vi "CM-TDT-Save config.vi"(0 "configuration file path":path=path "C:/PXI Connections.txt", 5 "Tables":cluster{"Table":T1[]}[](array[cluster]), 9 "Endpoints":cluster{"Items":string[]}[](array[cluster]), 11 "error in (no error)":errorcluster) -> (15 "error out":errorcluster)   [LabVIEW 2015]
uses:
  Type Defs/CM-Connection.ctl
  <vilib>/Utility/config.llb/Write Key (String).vi
  <vilib>/Utility/config.llb/NI_LVConfig.lvlib
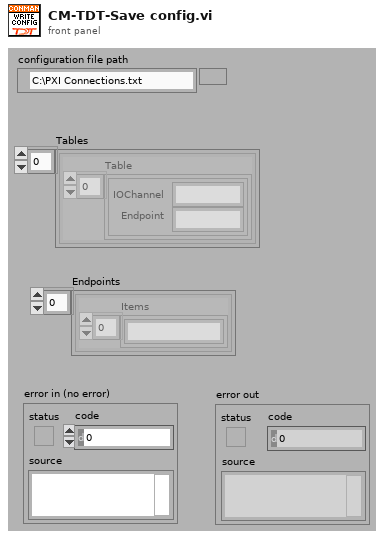
[diagram p1: front panel]
types:
  T1 = typedef "CM-Connection.ctl" = cluster{"IOChannel":string, "Endpoint":string}
  T2 = typedef "NI_LVConfig.lvlib/Config Data RefNum.ctl" = refnum<k1>
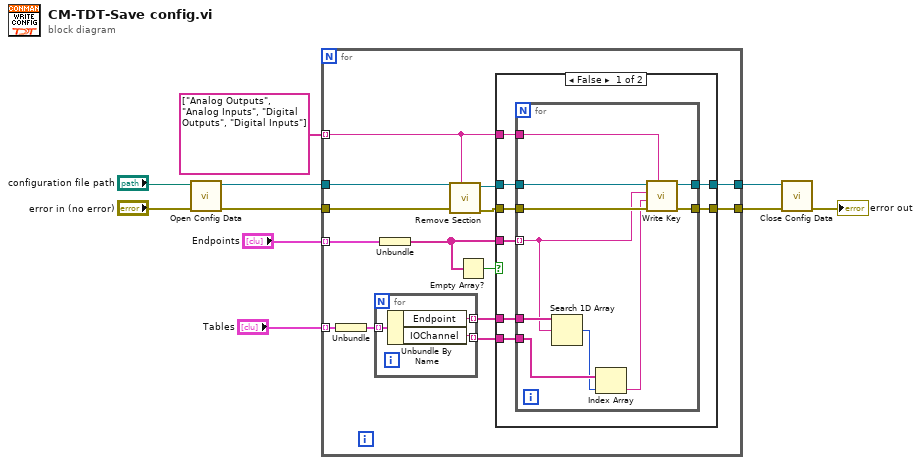
[diagram p0: block diagram]
diagram:
  n1 = call <vilib>:"Open Config Data.vi"("error in (no error)"="error in (no error)", "configuration file path"="configuration file path") -> ("error out"=w5:errorcluster, "refnum"=w6:T2)  [unwired: 7 in, 1 out]
  n2 = for {
    tunnel: [w24] -> w4
    tunnel: [w23] -> w3
    tunnel: string[] ["Analog Outputs", "Analog Inputs", "Digital Outputs", "Digital Inputs"] -> [w20] mode=indexing
    tunnel: w6 -> [w19]
    tunnel: w5 -> [w17]
    tunnel: "Endpoints" -> [w21] mode=indexing
    tunnel: "Tables" -> [w15] mode=indexing
    n3 = Unbundle(w15) -> ("Table"=w11:T1[])
    n4 = for {
      tunnel: w11 -> [w47] mode=indexing
      tunnel: [w46] -> w14 mode=indexing
      tunnel: [w45] -> w13 mode=indexing
      n5 = Unbundle By Name(w47) -> ("Endpoint"=w46:string, "IOChannel"=w45:string)
    }
    n6 = Unbundle(w21) -> ("Items"=w12:string[])
    n7 = call <vilib>:"Remove Section.vi"("section"=w20, "error in (no error)"=w17, "refnum"=w19) -> ("error out"=w16:errorcluster, "refnum out"=w18:T2)  [unwired: 6 in, 1 out]
    n8 = Empty Array?(array=w12) -> (empty?=w22:bool)
    n9 = case shown="False" w22 {
      tunnel: w14 -> [w32 _]
      tunnel: w18 -> [w31 w44]
      tunnel: w16 -> [w30 w43]
      tunnel: w12 -> [w29 _]
      tunnel: [w28 w44] -> w24
      tunnel: [w27 w43] -> w23
      tunnel: w20 -> [w26 _]
      tunnel: w13 -> [w25 _]
      frame False {
        n10 = for {
          tunnel: w29 -> [w37] mode=indexing
          tunnel: w32 -> [w42]
          tunnel: w31 -> [w41]
          tunnel: [w39] -> w28
          tunnel: w30 -> [w40]
          tunnel: [w38] -> w27
          tunnel: w26 -> [w36]
          tunnel: w25 -> [w35]
          n11 = Search 1D Array(1D array=w42, element=w37) -> (index of element=w34:i32)  [unwired: 1 in]
          n12 = Index Array(array=w35, index=w34) -> (element=w33:string)
          n13 = call-poly <vilib>:"Write Key.vi"("section"=w36, "error in (no error)"=w40, "value"=w33, "key"=w37, "refnum"=w41) -> ("error out"=w38:errorcluster, "refnum out"=w39:T2)  [unwired: 4 in, 1 out]
        }
      }
      frame True {
      }
    }
  }
  n14 = call <vilib>:"Close Config Data.vi"("error in (no error)"=w3, "refnum"=w4) -> ("error out"=→"error out":errorcluster)  [unwired: 8 in, 1 out]
